vi "Core Execute.vi"(8 "error in (no error)":errorcluster, 11 "CIFTemplateNode in":refnum<class "CIFCorePlugin.lvclass">) -> (0 "error out":errorcluster, 3 "CIFTemplateNode out":refnum<class "CIFCorePlugin.lvclass">)   [LabVIEW 2021, in "CIFCorePlugin.lvclass"]
uses:
  CIFCorePlugin.lvclass
  CIFCorePlugin.lvclass/CIFCorePlugin.ctl
  Typedef/Energized States.ctl
  CIFUtilities/CIFClocks/Core/Get Time.vi
  CIFUtilities/CIFClocks/Time Conversion/LabVIEW Time to UTC Time.vi
  CIFUtilities/CIFClocks/SubVIs/Add Error.vi
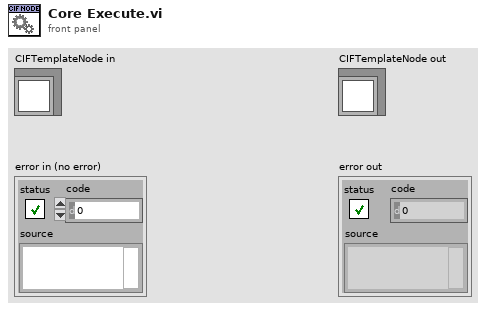
[diagram p1: front panel]
types:
  T1 = typedef "CIFCorePlugin.lvclass/Energized States.ctl" = enum16{"Listen", "Prepare", "Execute", "Housekeep", "Cleanup", "Destroy"}
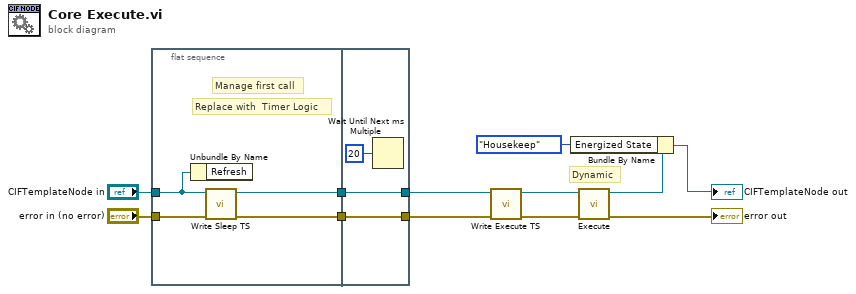
[diagram p0: block diagram]
diagram:
  # "Dynamic"
  n1 = flat-sequence {
    tunnel: "CIFTemplateNode in" -> [w13]
    tunnel: "error in (no error)" -> [w16]
    tunnel: [w15] -> w2
    tunnel: [w14] -> w1
    tunnel: [w18] -> w3
    tunnel: [w19] -> w4
    tunnel: w2 -> [w19]
    tunnel: w1 -> [w18]
    frame #0 {
      # "Manage first call"
      # "Replace with  Timer Logic"
      n2 = Unbundle By Name(w13) -> ()  [unwired: 1 out]
      n3 = call "Write Sleep TS.vi"("error in (no error)"=w16, "CIFCorePlugin in"=w13) -> ("error out"=w14:errorcluster, "CIFCorePlugin out"=w15:refnum<class "CIFCorePlugin.lvclass">)  [unwired: 8 in]
    }
    frame #1 {
      n4 = Wait Until Next ms Multiple(millisecond multiple=u32 20) -> ()  [unwired: 1 out]
    }
  }
  n5 = call "Write Execute TS.vi"("error in (no error)"=w3, "CIFCorePlugin in"=w4) -> ("error out"=w11:errorcluster, "CIFCorePlugin out"=w10:refnum<class "CIFCorePlugin.lvclass">)  [unwired: 8 in]
  n6 = call-dynamic "Execute.vi"("error in (no error)"=w11, "CIFTemplateNode in"=w10) -> ("error out"=→"error out":errorcluster, "CIFTemplateNode out"=w8:refnum<class "CIFCorePlugin.lvclass">)  [unwired: 8 in]
  n7 = Bundle By Name(cluster=w8, "Energized State"=Energized_States."Housekeep") -> (→"CIFTemplateNode out":refnum<class "CIFCorePlugin.lvclass">)
